vi "Create Column Definitions.vi"(8 "error in (no error)":errorcluster, 10 "Column":T1={"name"="", "caption"="", "datatype"=enum."string", "Params"="", "AutoSizeMode"=1, "FillWeight"=100.0, "MinWidth"=50, "tooltip"=""} {"MinWidth" min=2 step=1; "AutoSizeMode" items=["None"=1, "ColumnHeader"=2, "AllCellsExceptHeader"=4, "AllCells"=6, "DisplayedCellsExceptHeader"=8, "DisplayedCells"=10, "Fill"=16]; "FillWeight" min=1 max=100}) -> (0 "error out":errorcluster, 3 "GridColumn out":refnum<class "GridColumn.lvclass">)   [LabVIEW 2020, in "DataGrid.lvlib" / "GridColumn.lvclass"]
doc: "Based on the column inputs, the settings are applied to the .net TABLE column."
uses:
  GridColumn.lvclass
  ColumnDefinition.ctl
  ColumnType.ctl
  GridColumn.lvclass/GridColumn.ctl
  Write Name.vi
  Write datatype.vi
  Write Params.vi
  Write AutoSizeMode.vi
  Write Caption.vi
  Write Tooltip.vi
  Write FillWeight.vi
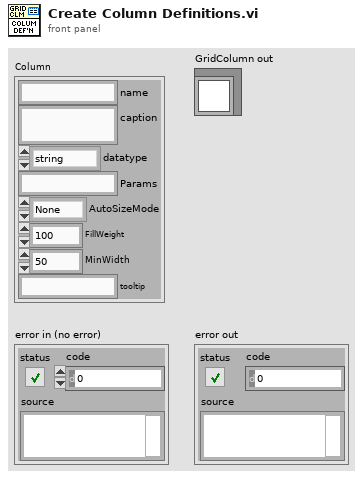
[diagram p1: front panel]
types:
  T1 = typedef "DataGrid.lvlib/GridColumn.lvclass/ColumnDefinition.ctl" = cluster{"name":string, "caption":string, "datatype":T2, "Params":string, "AutoSizeMode":i32, "FillWeight":sgl, "MinWidth":u32, "tooltip":string}
  T2 = typedef "DataGrid.lvlib/GridColumn.lvclass/ColumnType.ctl" = enum16{"string", "image", "check", "numeric", "timestamp", "button", "combo", "link"}
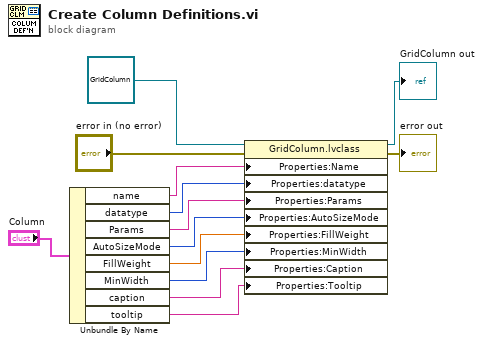
[diagram p0: block diagram]
diagram:
  n1 = Unbundle By Name("Column") -> ("name"=w10:string, "datatype"=w5:T2, "Params"=w11:string, "AutoSizeMode"=w12:i32, "FillWeight"=w13:sgl, "MinWidth"=w4:u32, "caption"=w2:string, "tooltip"=w1:string)
  n2 = property class="GridColumn.lvclass"(reference=refnum<class "GridColumn.lvclass"> refnum ("GridColumn in"), error in="error in (no error)", "Properties:Name"=w10, "Properties:datatype"=w5, "Properties:Params"=w11, "Properties:AutoSizeMode"=w12, "Properties:FillWeight"=w13, "Properties:MinWidth"=w4, "Properties:Caption"=w2, "Properties:Tooltip"=w1) -> (reference out=→"GridColumn out":refnum<class "GridColumn.lvclass">, error out=→"error out":errorcluster)
